vi "Send Current Settings.vi"(8 "error in (no error)":errorcluster, 11 "N5745A in":refnum<class "5745A.lvclass">) -> (0 "error out":errorcluster, 3 "N5745A out":refnum<class "5745A.lvclass">)   [LabVIEW 2018, in "5745A.lvlib" / "5745A.lvclass"]
doc: "This method is used to send tthe current setting to the N5745A Power Supply. It also enables the Over Current Protection (OCP)."
uses:
  5745A.lvclass
  builds/Power_Supply.lvlibp/Power Supply.lvclass
  C:/Users/Ron.Dexter.LUMINARTECH/Desktop/builds/Power_Supply.lvlibp/Power Supply.lvclass
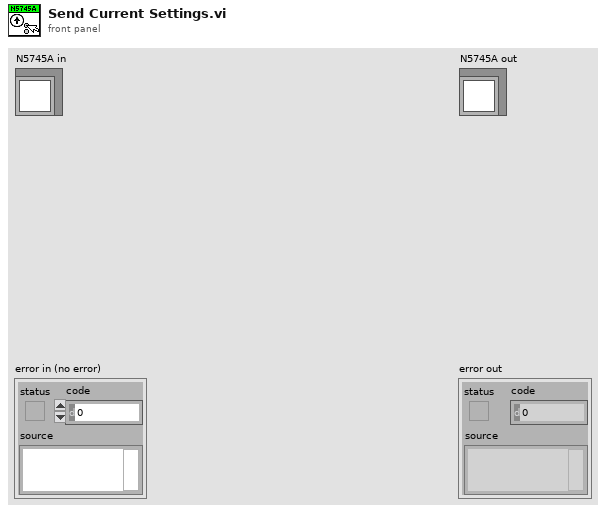
[diagram p1: front panel]
types:
  T1 = typedef "Power_Supply.lvlibp/Supply Settings.ctl" = cluster{"Voltage":dbl, "Current":dbl, "Output":bool}
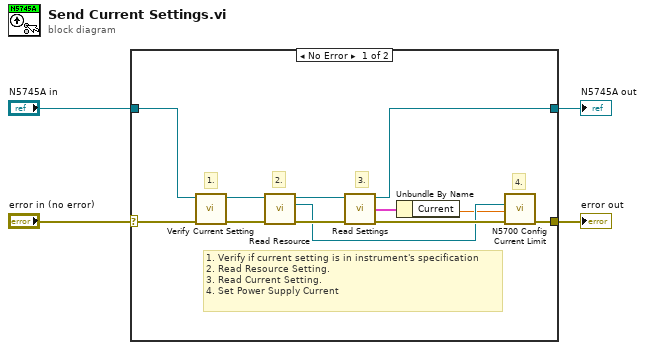
[diagram p0: block diagram]
diagram:
  n1 = case shown="No Error" "error in (no error)" {
    selector: "error in (no error)" -> [w14 w18]
    tunnel: [w5 w18] -> w3
    tunnel: [w11 w17] -> w1
    tunnel: "N5745A in" -> [w16 w17]
    frame No Error {
      # "3."
      # "2."
      # "1. Verify if current setting is in instrument's specification\n2. Read Resource Setting.\n3. Read Current Setting.\n4. Set Power Supply Current"
      # "4."
      # "1."
      n2 = call "Verify Current Setting.vi"("error in (no error)"=w14, "N5745A in"=w16) -> ("error out"=w13:errorcluster, "N5745A out"=w15:refnum<class "5745A.lvclass">)  [unwired: 8 in]
      n3 = call "Read Resource.vi"("error in"=w13, "Power Supply in"=w15) -> ("error out"=w10:errorcluster, "Resource"=w8:refnum<visa-resource-name>, "Power Supply out"=w12:refnum<class "5745A.lvclass">)  [unwired: 7 in]
      n4 = call "Read Settings.vi"("error in (no error)"=w10, "Power Supply in"=w12) -> ("error out"=w9:errorcluster, "Settings"=w7:T1, "Power Supply out"=w11:refnum<class "5745A.lvclass">)  [unwired: 7 in]
      n5 = Unbundle By Name(w7) -> ("Current"=w6:dbl)
      n6 = call <instrlib>:"N5700 Config Current Limit.vi"("error"=w9, "Current Limit"=w6, "VISA"=w8) -> ("error out"=w5:errorcluster)  [unwired: 4 in, 1 out]
    }
    frame Error {
    }
  }
  "error out" <- w3
  "N5745A out" <- w1
